vi "myRIO v1.0 Configure PWM.vi"(8 "error in (no error)":errorcluster, 9 "PWM Configuration":T4, 10 "PWM Channel":T1, 11 "myRIO Ref In":T2) -> (0 "error out":errorcluster, 2 "Max Counter Value":u16, 3 "Actual Frequency (Hz)":dbl)   [LabVIEW 2021]
uses:
  <vilib>/myRIO/Common/Instrument Driver Framework/myRIO v1.0/PWM/typedefs/PWM Configuration v1.0.ctl
  <vilib>/myRIO/Common/Instrument Driver Framework/Utilities/typedefs/myRIO v1.0 Reference.ctl
  <vilib>/myRIO/Common/Instrument Driver Framework/Utilities/typedefs/Generic FPGA Reference.ctl
  <vilib>/myRIO/Common/Instrument Driver Framework/myRIO v1.0/PWM/typedefs/PWM Channels Enum.ctl
  <vilib>/myRIO/Common/Instrument Driver Framework/myRIO v1.0/PWM/typedefs/PWM Channels FPGA Reference.ctl
  <vilib>/myRIO/Common/Instrument Driver Framework/Utilities/vis/Calculate Clock Settings.vi
  <vilib>/myRIO/Common/Instrument Driver Framework/Utilities/vis/Calculate TOP (Phase Correct Mode).vi
  <vilib>/myRIO/Common/Instrument Driver Framework/Utilities/vis/Calculate TOP (Normal Mode).vi
  <vilib>/myRIO/Common/Instrument Driver Framework/Utilities/vis/Calculate Frequency (Phase Correct Mode).vi
  <vilib>/myRIO/Common/Instrument Driver Framework/Utilities/vis/Calculate Frequency (Normal Mode).vi
  <vilib>/rvi/errors/niLvFpgaAdjustHostInterfaceError.vi
  <vilib>/rvi/interface/nirviReadWriteControl/nirviReadWriteControl.xnode
  <vilib>/rvi/interface/Simulation/niFpgaSimulationCallBeginRW.vi
  NiFpgaLv.dll
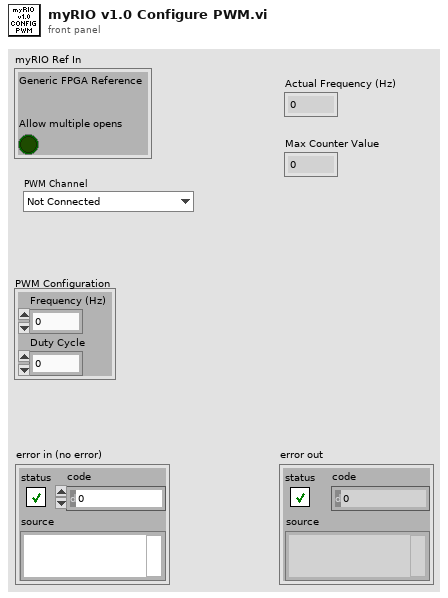
[diagram p1: front panel]
types:
  T1 = typedef "PWM Channels Enum.ctl" = enum16{"Not Connected", "C/PWM0", "C/PWM1", "A/PWM0", "A/PWM1", "A/PWM2", "A/PWM3", "A/PWM4", "A/PWM5", "A/PWM6", "A/PWM7", "A/PWM8", "A/PWM9", "A/PWM10", "A/PWM11", "A/PWM12", "A/PWM13", "A/PWM14", "A/PWM15", "A/PWM16", "A/PWM17", "A/PWM18", "A/PWM19", "B/PWM0", "B/PWM1", "B/PWM2", "B/PWM3", "B/PWM4", "B/PWM5", "B/PWM6", "B/PWM7", "B/PWM8", "B/PWM9", "B/PWM10", "B/PWM11", "B/PWM12", "B/PWM13", "B/PWM14", "B/PWM15", "B/PWM16", "B/PWM17", "B/PWM18", "B/PWM19", "PWM/PWM0", "PWM/PWM1", "PWM/PWM2", "PWM/PWM3", "PWM/PWM4", "PWM/PWM5", "PWM/PWM6", "PWM/PWM7", "PWM/PWM8", "PWM/PWM9"}
  T2 = typedef "myRIO v1.0 Reference.ctl" = cluster{"Generic FPGA Reference":T3, "Allow multiple opens":bool}
  T3 = typedef "Generic FPGA Reference.ctl" = refnum<k20>
  T4 = typedef "PWM Configuration v1.0.ctl" = cluster{"Frequency (Hz)":dbl, "Duty Cycle":dbl}
  T5 = typedef "PWM Channels FPGA Reference.ctl" = refnum<k20>
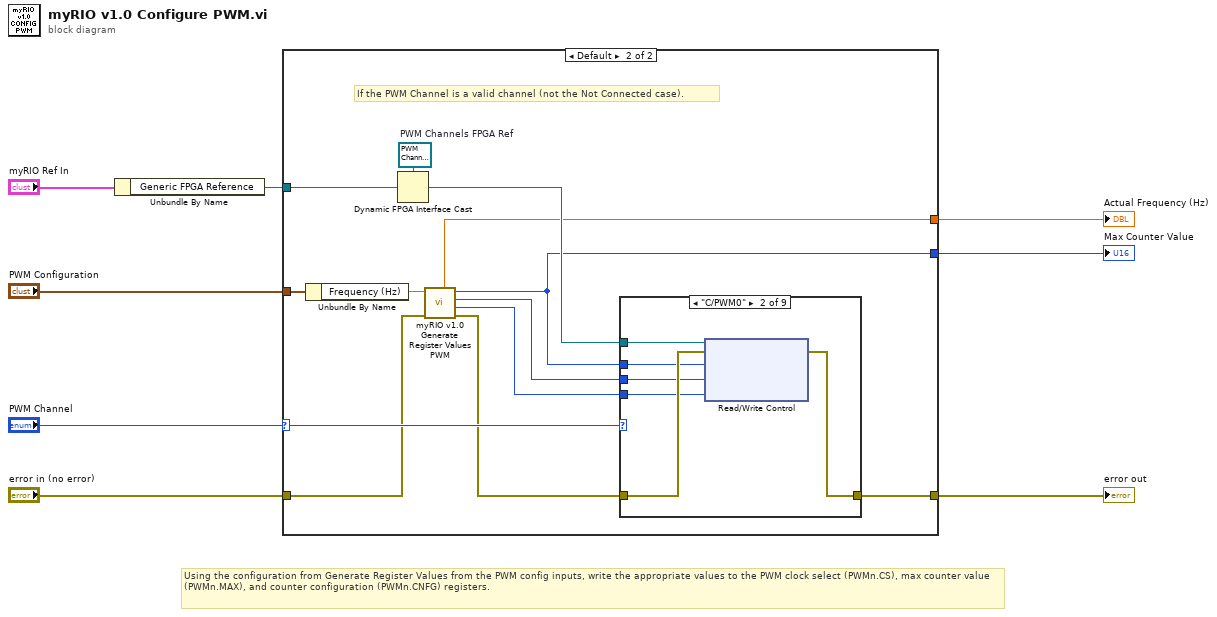
[diagram p0: block diagram]
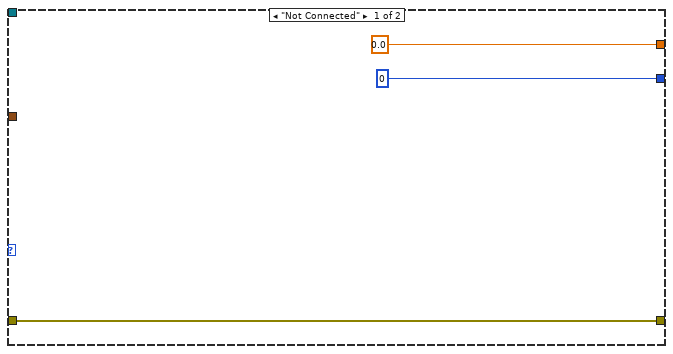
[diagram p2: hidden frame]
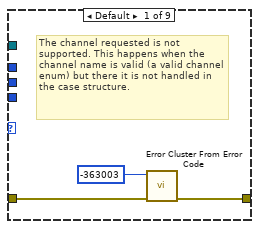
[diagram p3: hidden frame]
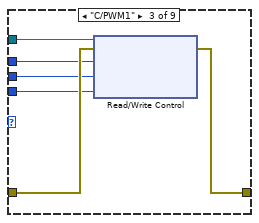
[diagram p4: hidden frame]
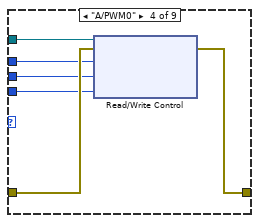
[diagram p5: hidden frame]
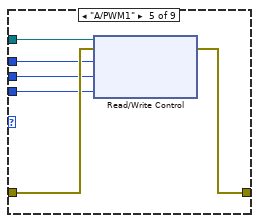
[diagram p6: hidden frame]
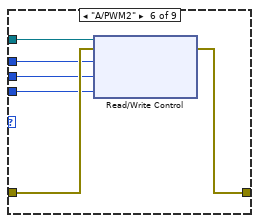
[diagram p7: hidden frame]
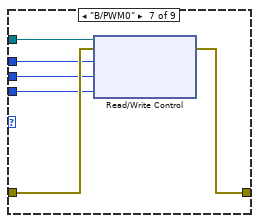
[diagram p8: hidden frame]
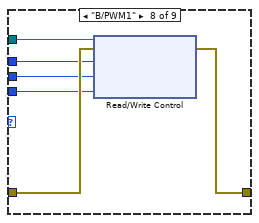
[diagram p9: hidden frame]
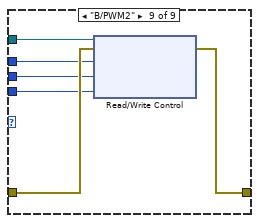
[diagram p10: hidden frame]
diagram:
  # "Using the configuration from Generate Register Values from the PWM config inputs, write the appropriate values to the PWM clock select (PWMn.CS), max counter value (PWMn.MAX), and counter configuration (PWMn.CNFG) registers."
  n1 = Unbundle By Name("myRIO Ref In") -> ("Generic FPGA Reference"=w1:T3)
  n2 = case shown="Default" "PWM Channel" {
    selector: "PWM Channel" -> [_ w20]
    tunnel: [w9 w22] -> w8
    tunnel: "PWM Configuration" -> [_ w13]
    tunnel: "error in (no error)" -> [w9 w15]
    tunnel: w1 -> [_ w21]
    tunnel: [u16 0 w18] -> w2
    tunnel: [0.0 ("Actual Frequency (Hz)") w19] -> w3
    frame "Not Connected" {
    }
    frame Default {
      w24 = T5 refnum  # PWM Channels FPGA Ref
      # "If the PWM Channel is a valid channel (not the Not Connected case)."
      n3 = Unbundle By Name(w13) -> ("Frequency (Hz)"=w12:dbl)
      n4 = Dynamic FPGA Interface Cast(Session In=w24, Type=w21) -> (Session Out=w23:T5)
      n5 = call <vilib>:"myRIO v1.0 Generate Register Values PWM.vi"("error in (no error)"=w15, "Frequency (Hz)"=w12) -> ("error out"=w14:errorcluster, "PWM.CS"=w16:u8, "PWM.CNFG"=w17:u8, "PWM.MAX"=w18:u16, "Actual Frequency (Hz)"=w19:dbl)  [unwired: 5 in]
      n6 = case shown="\"C/PWM0\"" w20 {
        tunnel: w14 -> [w25 w33 w39 w45 w51 w57 w63 w69 w75]
        tunnel: [w26 w32 w38 w44 w50 w56 w62 w68 w74] -> w22
        tunnel: w23 -> [_ w31 w37 w43 w49 w55 w61 w67 w73]
        tunnel: w18 -> [_ w29 w35 w41 w47 w53 w59 w65 w71]
        tunnel: w17 -> [_ w30 w36 w42 w48 w54 w60 w66 w72]
        tunnel: w16 -> [_ w28 w34 w40 w46 w52 w58 w64 w70]
        frame Default {
          # "The channel requested is not supported. This happens when the channel name is valid (a valid channel enum) but there it is not handled in the case structure."
          n7 = call <vilib>:"Error Cluster From Error Code.vi"("error in (no error)"=w25, "error code (0)"=-363003) -> ("error out"=w26:errorcluster)  [unwired: 7 in]
        }
        frame "C/PWM0" {
          n8 = xnode "Read/Write Control"("FPGA VI Reference In"=w31, "error in"=w33, "PWM.C_0.MAX"=w29, "PWM.C_0.CNFG"=w30, "PWM.C_0.CS"=w28) -> ("error out"=w32:errorcluster)  [unwired: 1 out]
        }
        frame "C/PWM1" {
          n9 = xnode "Read/Write Control"("FPGA VI Reference In"=w37, "error in"=w39, "PWM.C_1.MAX"=w35, "PWM.C_1.CNFG"=w36, "PWM.C_1.CS"=w34) -> ("error out"=w38:errorcluster)  [unwired: 1 out]
        }
        frame "A/PWM0" {
          n10 = xnode "Read/Write Control"("FPGA VI Reference In"=w43, "error in"=w45, "PWM.A_0.MAX"=w41, "PWM.A_0.CNFG"=w42, "PWM.A_0.CS"=w40) -> ("error out"=w44:errorcluster)  [unwired: 1 out]
        }
        frame "A/PWM1" {
          n11 = xnode "Read/Write Control"("FPGA VI Reference In"=w49, "error in"=w51, "PWM.A_1.MAX"=w47, "PWM.A_1.CNFG"=w48, "PWM.A_1.CS"=w46) -> ("error out"=w50:errorcluster)  [unwired: 1 out]
        }
        frame "A/PWM2" {
          n12 = xnode "Read/Write Control"("FPGA VI Reference In"=w55, "error in"=w57, "PWM.A_2.MAX"=w53, "PWM.A_2.CNFG"=w54, "PWM.A_2.CS"=w52) -> ("error out"=w56:errorcluster)  [unwired: 1 out]
        }
        frame "B/PWM0" {
          n13 = xnode "Read/Write Control"("FPGA VI Reference In"=w61, "error in"=w63, "PWM.B_0.MAX"=w59, "PWM.B_0.CNFG"=w60, "PWM.B_0.CS"=w58) -> ("error out"=w62:errorcluster)  [unwired: 1 out]
        }
        frame "B/PWM1" {
          n14 = xnode "Read/Write Control"("FPGA VI Reference In"=w67, "error in"=w69, "PWM.B_1.MAX"=w65, "PWM.B_1.CNFG"=w66, "PWM.B_1.CS"=w64) -> ("error out"=w68:errorcluster)  [unwired: 1 out]
        }
        frame "B/PWM2" {
          n15 = xnode "Read/Write Control"("FPGA VI Reference In"=w73, "error in"=w75, "PWM.B_2.MAX"=w71, "PWM.B_2.CNFG"=w72, "PWM.B_2.CS"=w70) -> ("error out"=w74:errorcluster)  [unwired: 1 out]
        }
      }
    }
  }
  "error out" <- w8
  "Actual Frequency (Hz)" <- w3
  "Max Counter Value" <- w2
